vi "Init_Logging.vi"(0 "Main Init VI path":path, 7 "App.Kind":T1(ring), 11 "error in (no error)":errorcluster) -> (15 "error out":errorcluster)   [LabVIEW 2019, in "Service.lvlib"]
uses:
  Service.lvlib
  <vilib>/Field R&D Services/Logger/Field_RnD_Services_Logger_Toolkit.lvlib
  <vilib>/Field R&D Services/Logger/Type Definitions/Configuration.ctl
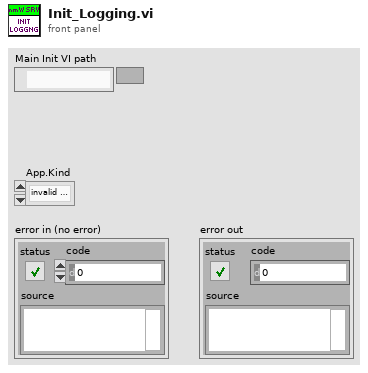
[diagram p1: front panel]
types:
  T1 = enum32{"invalid app kind", "Development System", "Run Time System", "Student Edition", "Embedded LabVIEW", "Evaluation", "Custom"}
  T2 = typedef "Field_RnD_Services_Logger_Toolkit.lvlib/Configuration.ctl" = cluster{"Delimiter":string, "Enable Calendar Tree":bool, "File Extension":string, "Maximum File Count":i32, "Maximum File Size":i64, "Prune All":bool, "Root Folder":path}
  T3 = typedef "Service.lvlib/AppData.ctl" = cluster{"MsgQ":refnum<queue>, "Stop?":bool, "zmq sessions":cluster{"Control_endpoint":string, "Instr_endpoint":string}, "control-loop":cluster{"fromUI-Q":refnum<queue>, "toUI":refnum<user-event>, "Control_endpoint":string}, "UI-loop":cluster{"evnt_ref":refnum<event-registration>}, "logging":cluster{"level":dbl, "verbosity":dbl, "path":string, "Listener_ID":string}}
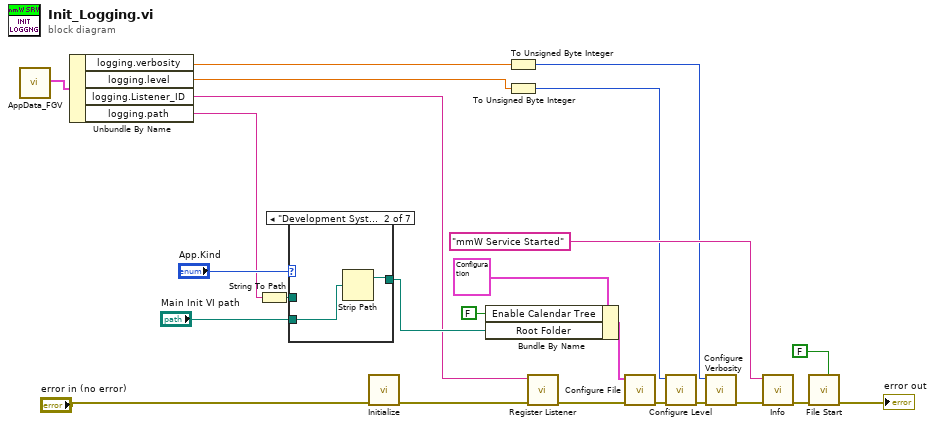
[diagram p0: block diagram]
diagram:
  n1 = call "AppData_FGV.vi"() -> ("AppData out"=w7:T3)  [unwired: 18 in, 1 out]
  n2 = Unbundle By Name(w7) -> ("logging.verbosity"=w4:dbl, "logging.level"=w3:dbl, "logging.Listener_ID"=w5:string, "logging.path"=w6:string)
  n3 = String To Path(string=w6) -> (path=w24:path)
  n4 = case shown="\"Development System\"" "App.Kind" {
    tunnel: [w25 w27 w28 w29 w30 w31 w32] -> w10
    tunnel: w24 -> [w25 _ w28 w29 w30 w31 w32]
    tunnel: "Main Init VI path" -> [_ w26 _ _ _ _ _]
    frame "invalid app kind", Default {
    }
    frame "Development System" {
      n5 = Strip Path(path=w26) -> (stripped path=w27:path)  [unwired: 1 out]
    }
    frame "Run Time System" {
    }
    frame "Student Edition" {
    }
    frame "Embedded LabVIEW" {
    }
    frame "Evaluation" {
    }
    frame "Custom" {
    }
  }
  n6 = call <vilib>:"Initialize.vi"("Error In"="error in (no error)") -> ("Error Out"=w20:errorcluster)  [unwired: 10 in]
  n7 = Bundle By Name(cluster=T2 {"Delimiter"=",", "Enable Calendar Tree"=TRUE, "File Extension"="csv", "Maximum File Count"=5, "Maximum File Size"=15728640, "Prune All"=FALSE, "Root Folder"=path ""} ("Configuration"), "Enable Calendar Tree"=FALSE, "Root Folder"=w10) -> (w21:T2)
  n8 = To Unsigned Byte Integer(number=w4) -> (unsigned 8bit integer=w1:u8)
  n9 = To Unsigned Byte Integer(number=w3) -> (unsigned 8bit integer=w2:u8)
  n10 = call <vilib>:"Register Listener.vi"("Error In"=w20, "Listener ID"=w5) -> ("Error Out"=w19:errorcluster)  [unwired: 9 in]
  n11 = call <vilib>:"Configure File.vi"("Error In"=w19, "Configuration"=w21) -> ("Error Out"=w18:errorcluster)  [unwired: 9 in]
  n12 = call <vilib>:"Configure Level.vi"("Error In"=w18, "Level"=w2) -> ("Error Out"=w17:errorcluster)  [unwired: 9 in]
  n13 = call <vilib>:"Configure Verbosity.vi"("Error In"=w17, "Verbosity"=w1) -> ("Error Out"=w15:errorcluster)  [unwired: 9 in]
  n14 = call <vilib>:"Info.vi"("Error In"=w15, "Message"="mmW Service Started") -> ("Error Out"=w14:errorcluster)  [unwired: 9 in]
  n15 = call <vilib>:"File Start.vi"("Run in Background"=FALSE, "Error In"=w14) -> ("Error Out"=→"error out":errorcluster)  [unwired: 9 in]
